vi "Dashboard Main.vi"() -> ()   [LabVIEW 2017]
uses:
  <vilib>/Utility/miscctls.llb/LVRowAndColumnTypeDef.ctl
  <vilib>/event_ctls.llb/eventvkey.ctl
  <vilib>/Rock Robotics/Network Tables/NT Read Numeric Array.vi
  <vilib>/Rock Robotics/WPI/Dashboard/WPI_DashboardLogging Global.vi
  <vilib>/Rock Robotics/Network Tables/NT Write Boolean.vi
panel:
  in  "Camera Settings Right":T1={"Frame Rate"=30, "Compression"=30, "Size"=1, "DB Camera Config"=FALSE} {"Frame Rate" scale=1.0..30.0; "Compression" scale=100.0..-1.0; "Size" items=["640x480", "320x240", "160x120"]}
  in  "Camera Name Right":string(combo)="No Camera Selection"
  out "Camera Info":cluster{"Mbps LED":bool, "Mbps":dbl, "fps":dbl} {"fps" format="%#.1g"; "Mbps" format="%#.1g"}
  in  "Camera Settings":T1={"Frame Rate"=30, "Compression"=30, "Size"=1, "DB Camera Config"=FALSE} {"Frame Rate" scale=1.0..30.0; "Compression" scale=100.0..-1.0; "Size" items=["640x480", "320x240", "160x120"]}
  in  "TCP":refnum<k5>
  in  "Rec Mode":enum32{"Stop", "Record", "Playback"}(radio)
  out "Robot IP":string
  out "Image Message":string="Timeout in Camera Communications"
  in  "Dashboard Tab":T2(tab)
  out "Game Data":string
  in  "Select test":string(combo)="with_delay"
  out "NT Connection":bool
  out "MotorChart R":cluster{"Numeric":dbl, "Numeric":dbl}(graph)
  out "MotorChart L":cluster{"Numeric":dbl, "Numeric":dbl}(graph)
  out "MotorSliders R":cluster{"MotorSlide1":dbl, "MotorSlide2":dbl} {"MotorSlide2" scale=-1.0..1.0 scale format="%#_2e"; "MotorSlide1" scale=-1.0..1.0 scale format="%#_2e"}
  out "MotorSliders L":cluster{"MotorSlide1":dbl, "MotorSlide2":dbl} {"MotorSlide2" scale=-1.0..1.0 scale format="%#_2e"; "MotorSlide1" scale=-1.0..1.0 scale format="%#_2e"}
  out "JS1 Z":dbl(slide) scale=-1.0..1.0 scale format="%#_2e"
  out "JS1 Graph":cluster{"X":dbl, "Y":dbl}[](graph)
  out "JS1 Buttons":T3
  out "JS2 Z":dbl(slide) scale=-1.0..1.0 scale format="%#_2e"
  out "JS2 Graph":cluster{"X":dbl, "Y":dbl}[](graph)
  out "JS2 Buttons":T3
  out "Mode":T4(ring)=enum."Auto Disabled"
  out "Camera Image Right":T5(plugin-control)
  in  "DB/String 9":string
  in  "DB/String 8":string
  in  "DB/String 7":string
  in  "DB/String 6":string
  in  "DB/String 5":string
  in  "DB/String 4":string
  in  "DB/String 3":string
  in  "DB/String 2":string
  in  "DB/String 1":string
  in  "DB/String 0":string
  in  "DB/Slider 0":dbl(slide) scale=0.0..5.0
  in  "DB/Slider 1":dbl(slide) scale=0.0..5.0
  in  "DB/Slider 2":dbl(slide) scale=0.0..5.0
  in  "DB/Slider 3":dbl(slide) scale=0.0..5.0
  out "DB/LED 3":bool
  out "DB/LED 2":bool
  out "DB/LED 1":bool
  out "DB/LED 0":bool
  in  "DB/Button 3":bool
  in  "DB/Button 2":bool
  in  "DB/Button 1":bool
  in  "DB/Button 0":bool caption="New Name"
  in  "Position":string(combo)="L"
  in  "A second driver":bool
  in  "Select Auto":string(combo)="with_delay"
  in  "Test Slider":dbl(slide) scale=0.0..100.0 scale format="%#_3g"
  in  "On/Off":bool caption="Solenoid"
  in  "Test Name":u16(ring) items=["Select the test to run..."]
  in  "Test Tree":string(tree)
  in  "Motor":cluster{"Value":dbl, "Enable":bool} {"Value" scale=-1.0..1.0 scale format="%#_3g"}
  out "Progress":T6 {"Test Progress" scale=0.0..100.0}
  in  "Rev/Fwd":cluster{"Forward":bool, "Reverse":bool}
  in  "Test Ring":u16(ring) items=["Monochrome", "Color"]
  out "Cmd Status":string
  in  "Execute Command":bool
  in  "Command Params":string[][](table)
  in  "Command Selection":i32(listbox)
  in  "CheckList":i32(listbox)
  out "Tree":string(tree)
  out "Camera Image":T5(plugin-control)
  out "Background":bool
  in  "Camera Name":string(combo)="Camera"
  # "HW"
  # "HW"
  # "Front"
  # "Joysticks"
  # "Left"
  # "Right"
  # "Back"
  # "This string shows the position of the switch and the scale,\nthe first letter is our switch,the second is the scale,\nand the last one is OPFOR's switch."
  # "This tab is a great place for autonomous settings and robot-specific values.\nPlace controls and indicators inside this tab and match name to\nDashboard Variables on robot. You can also delete this comment."
  # "This auto selector is not used any more,\nbecause the combo button seldom works."
  # "If you press that, the teleop will\nchange to the dual driver mode.\n(DISABLED NOW,always in dual mode)"
  # "Which tells you the actual position\nof the robot when you change it\nwith your other alliance member."
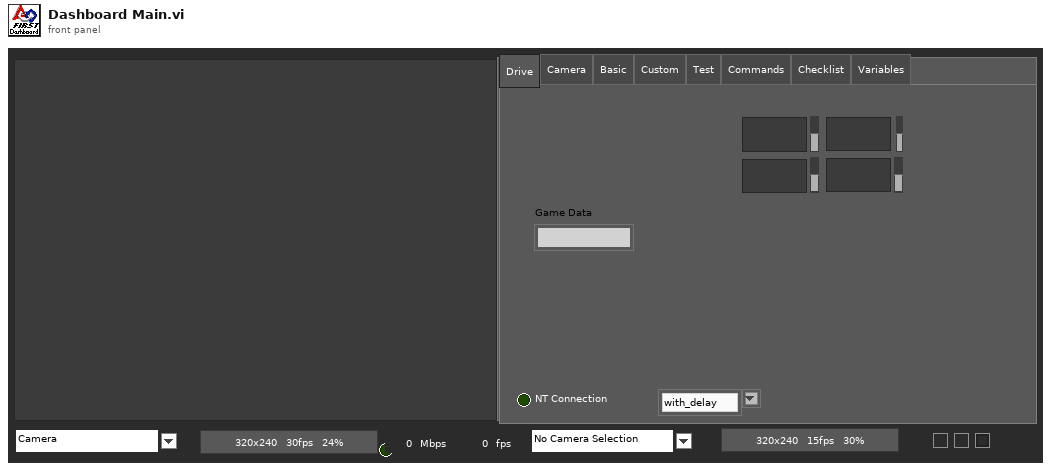
[diagram p1: front panel]
types:
  T1 = cluster{"Frame Rate":i32, "Compression":i32, "Size":u16, "DB Camera Config":bool}
  T2 = enum32{"Drive", "Camera", "Basic", "Custom", "Test", "Commands", "Checklist", "Variables"}
  T3 = cluster{bool, bool, bool, bool, bool, bool, bool, bool, bool, bool, bool, bool}
  T4 = enum8{"Tele-Op Disabled", "Tele-Op Enabled", "Auto Disabled", "Auto Enabled", "Test Disabled", "Test Enabled", "Disconnected", "No Code", "E-Stop"}
  T5 = typedef "IMAQ Image.ctl" = refnum<image>
  T6 = cluster{"Test Progress":u8, "Test Progress Text":string}
  T7 = cluster{"Save Path":path, "Interval (s)":dbl, "Keep":i32}
  T8 = typedef "Image Type" = u32
  T9 = cluster{"IDs":cluster{"RPC field ID":u16, "Unique ID":u16}, "String":string}
  T10 = cluster{"Error Strings":string, "Disable Counts":cluster{u16, u16}, "Rail Faults":cluster{u16, u16, u16}, "Robot IP":string, "DB Mode":u8, "Event Info":cluster{"Name":string, "Type":u8, "Number":u16, "Replay":u8}}
  T11 = cluster{"Storage":cluster{"Disk Free":u64, "RAM Block":u32, "RAM free":u32}, "CPU Utilization":cluster{"CPU % ISR":sgl, "CPU % Time Crit":sgl, "CPU % Timed Str":sgl, "CPU % High":sgl, "CPU % Above":sgl, "CPU % Normal":sgl, "CPU % Low":sgl}, "CAN":cluster{"% Bus Utilization":sgl, "Bus Off Cnt":u32, "TX_FIFO Full Cnt":u32, "Receive Error Cnt":u8, "Transmit Error Cnt":u8}, "HID":cluster{"HID Outputs":u32, "Rumble Low":u16, "Rumble High":u16}[]}
  T12 = cluster{"Status bits":cluster{"Test Mode":bool, "Autonomous":bool, "Enabled":bool, "Code Start":bool, "Brownout":bool, "Reserved 2":bool, "Reserved 3":bool, "E-Stop":bool}, "Code Trace":cluster{"Disabled":bool, "TeleOp":bool, "Auto":bool, "Test":bool}, "Controller Type":enum16{"unknown", "cRIO", "roboRio"}, "Code?":enum16{"unknown", "noCode", "code"}, "Battery V":dbl}
  T13 = cluster{"Control Bits":cluster{"TestMode":bool, "Autonomous":bool, "Enabled":bool, "FMS Present":bool, bool, bool, bool, "E-Stop":bool}, "Team Station ":u8, "Countdown":sgl, "Joystick Values":cluster{"Axes":dbl[], "Buttons":bool[], "POVs":i16[]}[]}
  T14 = cluster{"Axes":dbl[], "Buttons":bool[], "POVs":i16[]}[]
  T15 = cluster{"Axes":dbl[], "Buttons":bool[], "POVs":i16[]}
  T16 = cluster{"Buttons[0]":bool, "Buttons[1]":bool, "Buttons[2]":bool, "Buttons[3]":bool, "Buttons[4]":bool, "Buttons[5]":bool, "Buttons[6]":bool, "Buttons[7]":bool, "Buttons[8]":bool, "Buttons[9]":bool, "Buttons[10]":bool, "Buttons[11]":bool}
  T17 = cluster{"Camera Image":refnum<vi>, "Dashboard Tab":refnum<vi>, "Background":refnum<vi>, "Rec Mode":refnum<vi>, "Test Slider":refnum<vi>, "On/Off ":refnum<vi>, "Test Ring":refnum<vi>, "Rev/Fwd":refnum<vi>, "Test Name":refnum<vi>, "Motor":refnum<vi>, "Progress":refnum<vi>, "CheckList":refnum<vi>, "Tree":refnum<vi>, "Test Tree":refnum<vi>, "Command Params":refnum<vi>, "Command Selection":refnum<vi>, "Execute Command":refnum<vi>, "Cmd Status":refnum<vi>, "Camera Settings":refnum<vi>, "Camera Name":refnum<vi>, "Camera Info":refnum<vi>, "Camera Settings Right":refnum<vi>, "Camera Name Right":refnum<vi>, "Camera Image Right":refnum<vi>}
  T18 = cluster{"Camera Name":string, string, "Saved DB Images Info":cluster{"Save Path":path, "Interval (s)":dbl, "Keep":i32}}
  T19 = cluster{"Camera Name Right":string, string, "Saved DB Images Info":cluster{"Save Path":path, "Interval (s)":dbl, "Keep":i32}}
  T20 = cluster{"Operation":enum16{"Update", "Clear"}, "Color Box":u32}[]
  T21 = typedef "eventvkey.ctl" = enum16{"ASCII", "Enter", "Return", "Shift", "Ctrl", "Alt", "Cmd", "Opt", "Caps", "NumLock", "Clear", "Break", "Up", "Down", "Left", "Right", "Insert", "Delete", "Home", "End", "PageUp", "PageDown", "Escape", "Help", "Pause", "ScrollLock", "F1", "F2", "F3", "F4", "F5", "F6", "F7", "F8", "F9", "F10", "F11", "F12", "F13", "F14", "F15", "F16", "F17", "F18", "F19", "F20", "F21", "F22", "F23", "F24", "Play", "VolumeUp", "VolumeDown", "Mute", "Two Byte Char"}
  T22 = cluster{"Image Size":bool, "Image Type":bool, "Pixel Value":bool, "ROI Information":bool, "Zoom Factor":bool}
  T23 = cluster{"Operation":enum16{"Update", "Clear"}, "Color Box":u32}
  T24 = typedef "LVRowAndColumnTypeDef.ctl" = cluster{"Row":i32, "Column":i32}
  T25 = cluster{"Shift":bool, "Ctrl":bool, "Alt":bool, "Cmd":bool, "Opt":bool}
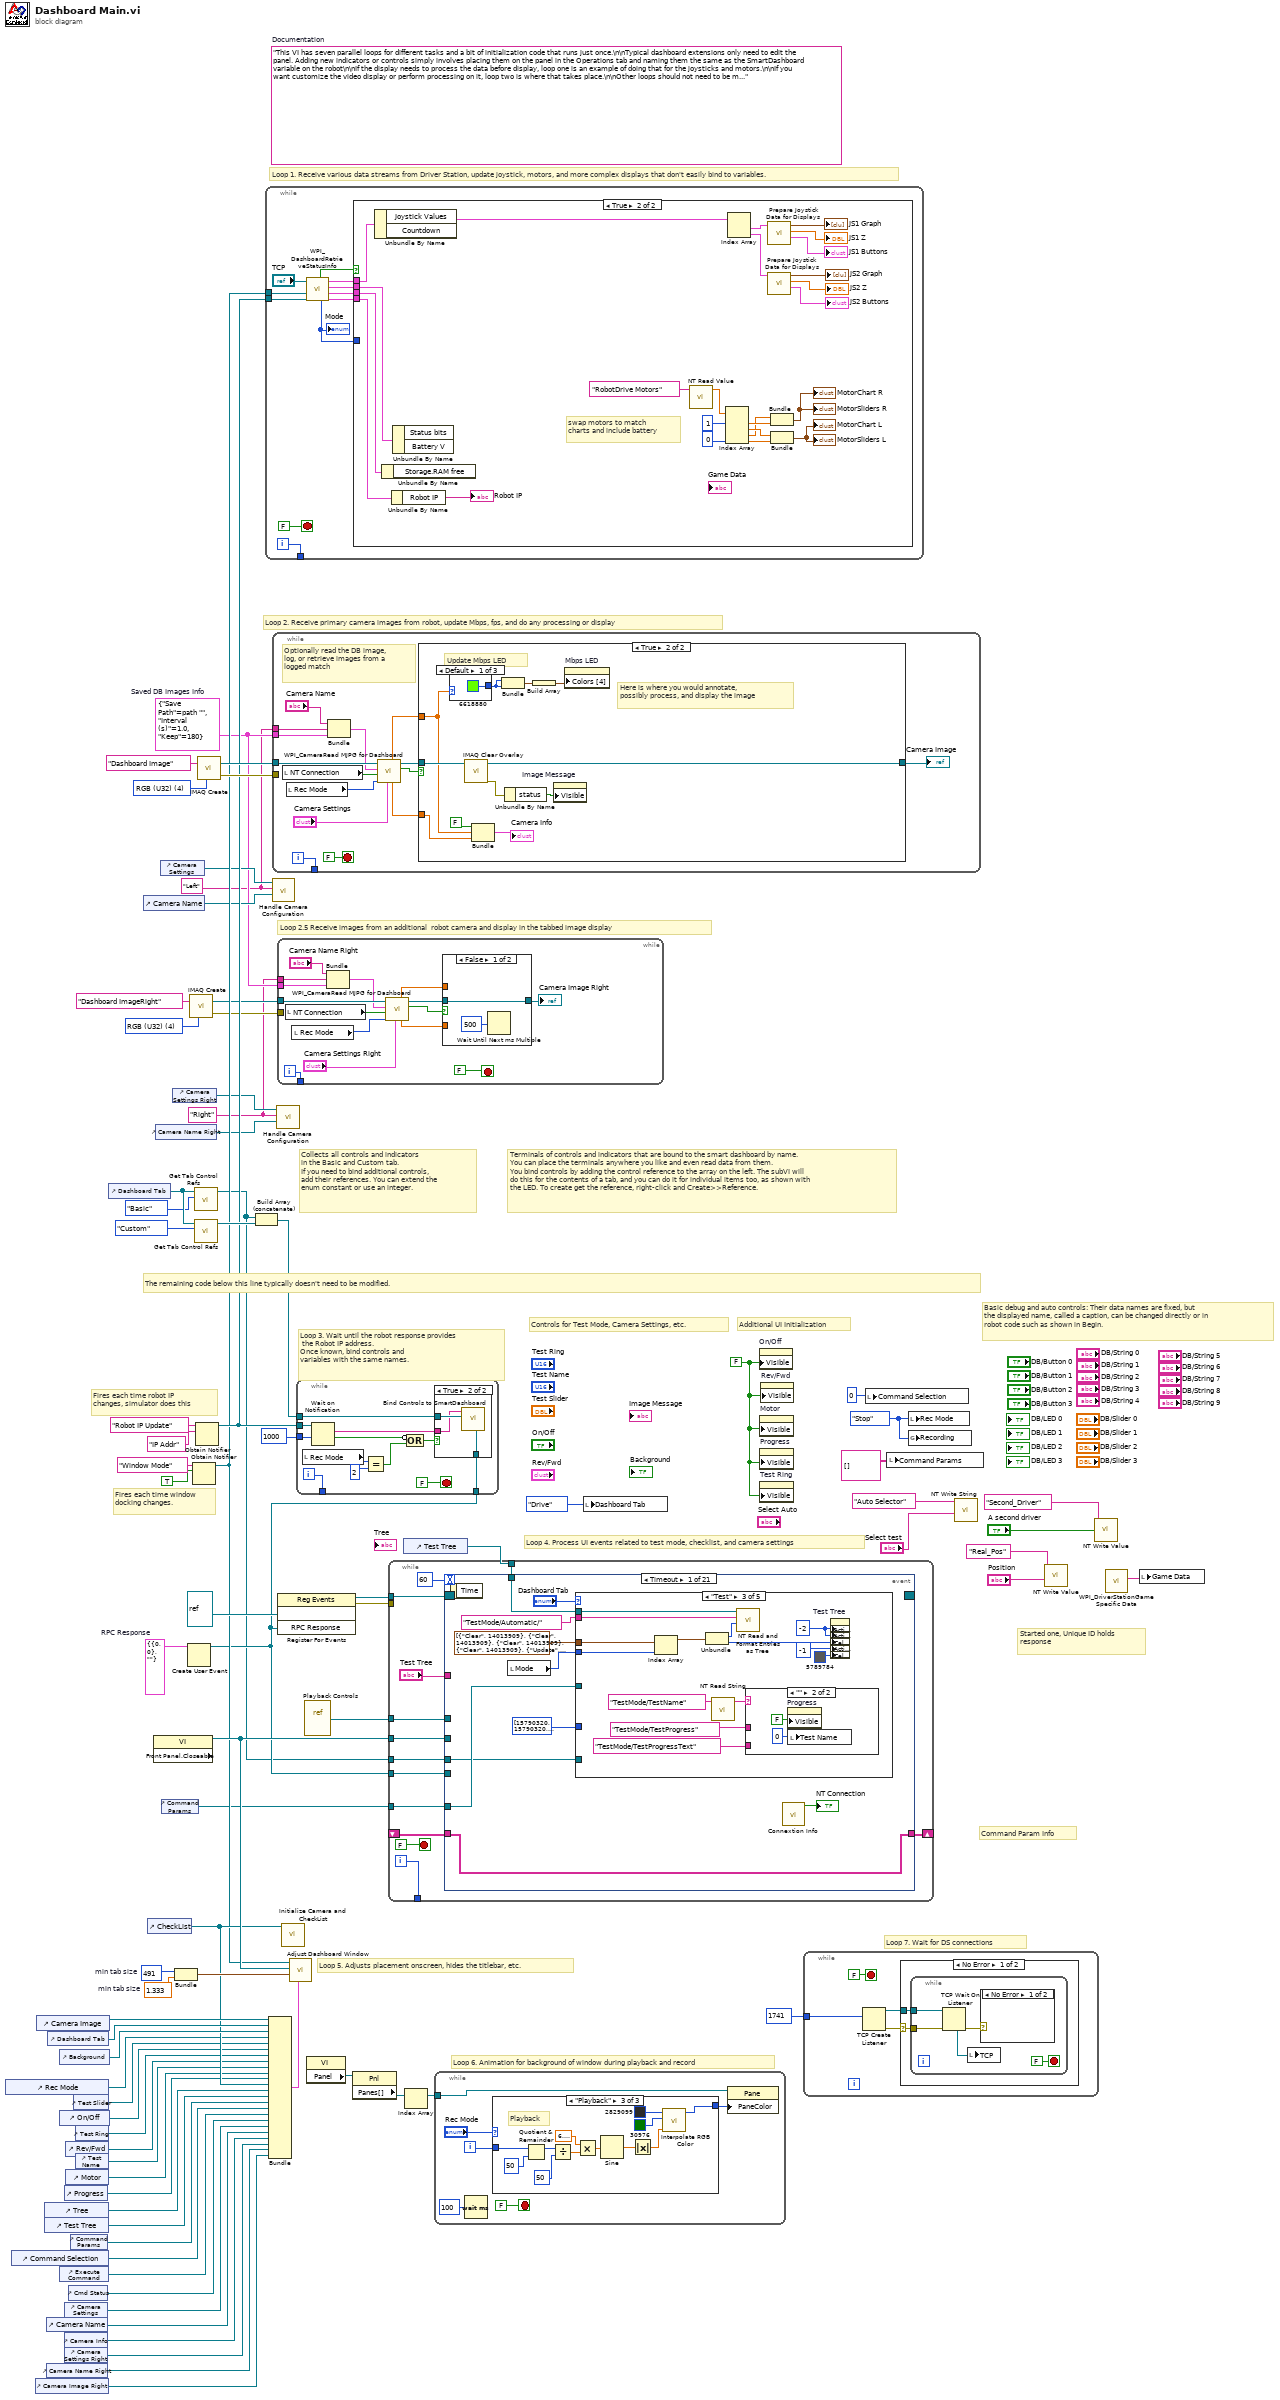
[diagram p0: block diagram]
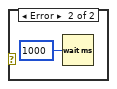
[diagram p3: hidden frame]
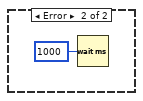
[diagram p4: hidden frame]
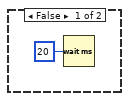
[diagram p5: hidden frame]
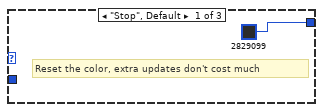
[diagram p6: hidden frame]
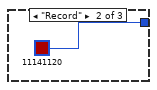
[diagram p7: hidden frame]
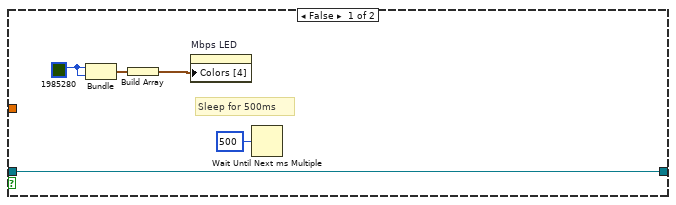
[diagram p9: hidden frame]
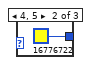
[diagram p10: hidden frame]
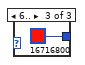
[diagram p11: hidden frame]
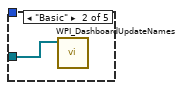
[diagram p13: hidden frame]
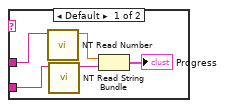
[diagram p14: hidden frame]
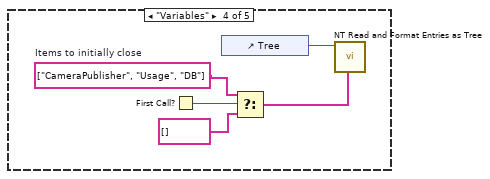
[diagram p15: hidden frame]
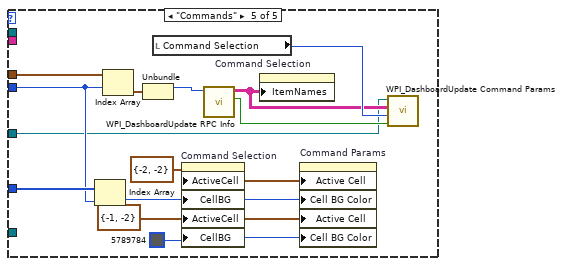
[diagram p16: hidden frame]
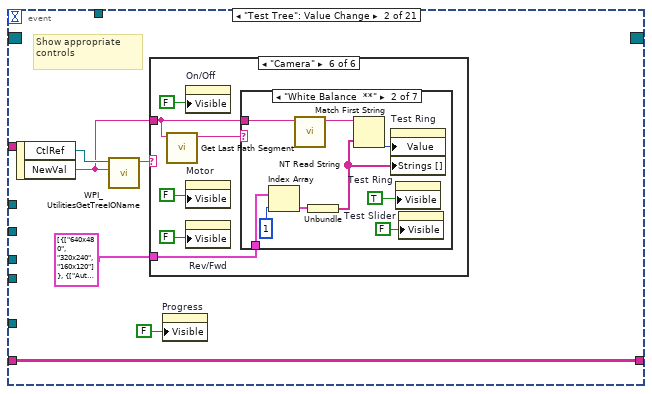
[diagram p17: hidden frame]
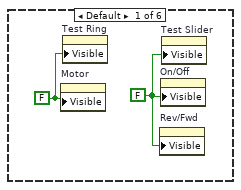
[diagram p18: hidden frame]
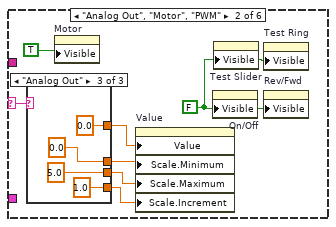
[diagram p19: hidden frame]
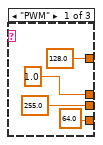
[diagram p20: hidden frame]
diagram:
  w9 = T7 {"Save Path"=path "", "Interval (s)"=1.0, "Keep"=180}  # Saved DB Images Info
  w8 = "Right"
  w7 = "Left"
  w19 = T8 4 items=["Grayscale (U8)", "Grayscale (I16)", "Grayscale (SGL)", "Complex (CSG)", "RGB (U32)", "HSL (U32)", "RGB (U64)"] ("Image Type")
  w34 = T9 {"IDs"={"RPC field ID"=0, "Unique ID"=0}, "String"=""}  # RPC Response
  w57 = 491  # min tab size
  w56 = 1.333  # min tab size
  w64 = enum32{"Stop", "Record", "Playback"}."Stop" ("Rec Mode")
  w41 = FALSE ("Visible")
  (unwired) "This VI has seven parallel loops for different tasks and a bit of initialization code that runs just once.\n\nTypical dashboard extensions only need to edit the panel. Adding new indicators or controls simply involves placing them on the panel in the Operations tab and naming them the same as the SmartDashboard variable on the robot\n\nIf the display needs to process the data before display, loop one is an example of doing that for the joysticks and motors.\n\nIf you want customize the video display or perform processing on it, loop two is where that takes place.\n\nOther loops should not need to be modified. They are pretty standard, and document the task they perform."  # Documentation
  w81 = T8 4 items=["Grayscale (U8)", "Grayscale (I16)", "Grayscale (SGL)", "Complex (CSG)", "RGB (U32)", "HSL (U32)", "RGB (U64)"] ("Image Type")
  # "Loop 2.5 Receive images from an additional  robot camera and display in the tabbed image display"
  # "Command Param Info"
  # "Started one, Unique ID holds\nresponse"
  # "Loop 7. Wait for DS connections"
  # "Basic debug and auto controls: Their data names are fixed, but\nthe displayed name, called a caption, can be changed directly or in\nrobot code such as shown in Begin."
  # "Controls for Test Mode, Camera Settings, etc."
  # "Additional UI Initialization"
  # "Loop 6. Animation for background of window during playback and record"
  # "Fires each time robot IP\nchanges, simulator does this"
  # "Fires each time window\ndocking changes."
  # "Collects all controls and indicators\nin the Basic and Custom tab.\nIf you need to bind additional controls,\nadd their references. You can extend the\nenum constant or use an integer."
  # "The remaining code below this line typically doesn't need to be modified."
  # "Loop 4. Process UI events related to test mode, checklist, and camera settings"
  # "Terminals of controls and indicators that are bound to the smart dashboard by name.\nYou can place the terminals anywhere you like and even read data from them.\nYou bind controls by adding the control reference to the array on the left. The subVI will\ndo this for the contents of a tab, and you can do it for individual items too, as shown with\nthe LED. To create get the reference, right-click and Create>>Reference."
  # "Loop 3. Wait until the robot response provides\n the Robot IP address.\nOnce known, bind controls and\nvariables with the same names."
  # "Loop 5. Adjusts placement onscreen, hides the titlebar, etc."
  # "Loop 1. Receive various data streams from Driver Station, update joystick, motors, and more complex displays that don't easily bind to variables."
  # "Loop 2. Receive primary camera images from robot, update Mbps, fps, and do any processing or display"
  n1 = control-ref of="Rec Mode"() -> (w47:refnum<vi>)
  n2 = control-ref of="Command Selection"() -> (w33:refnum<vi>)
  n3 = control-ref of="Camera Image Right"() -> (w12:refnum<vi>)
  n4 = control-ref of="Camera Image"() -> (w59:refnum<vi>)
  n5 = control-ref of="Tree"() -> (w51:refnum<vi>)
  n6 = control-ref of="Test Tree"() -> (w50:refnum<vi>)
  n7 = control-ref of="Camera Name"() -> (w24:refnum<vi>)
  n8 = control-ref of="Camera Name Right"() -> (w13:refnum<vi>)
  n9 = control-ref of="Dashboard Tab"() -> (w58:refnum<vi>)
  n10 = control-ref of="Execute Command"() -> (w35:refnum<vi>)
  n11 = control-ref of="Background"() -> (w54:refnum<vi>)
  n12 = control-ref of="On/Off"() -> (w45:refnum<vi>)
  n13 = control-ref of="Progress"() -> (w42:refnum<vi>)
  n14 = control-ref of="Camera Settings"() -> (w25:refnum<vi>)
  n15 = control-ref of="Camera Info"() -> (w23:refnum<vi>)
  n16 = control-ref of="Camera Settings Right"() -> (w14:refnum<vi>)
  n17 = control-ref of="Rev/Fwd"() -> (w43:refnum<vi>)
  n18 = control-ref of="Motor"() -> (w48:refnum<vi>)
  n19 = control-ref of="Cmd Status"() -> (w29:refnum<vi>)
  n20 = control-ref of="Command Params"() -> (w36:refnum<vi>)
  n21 = control-ref of="Test Slider"() -> (w46:refnum<vi>)
  n22 = control-ref of="Test Ring"() -> (w44:refnum<vi>)
  n23 = control-ref of="Test Name"() -> (w49:refnum<vi>)
  n24 = control-ref of="Dashboard Tab"() -> (w62:refnum<vi>)
  n25 = control-ref of="Camera Name"() -> (w26:refnum<vi>)
  n26 = control-ref of="CheckList"() -> (w52:refnum<vi>)
  n27 = property class="VI" props=["Front Panel.Closeable"]() -> (reference out=w63:refnum<vi>)  [unwired: 2 in, 2 out]
  n28 = control-ref of="Camera Name Right"() -> (w15:refnum<vi>)
  n29 = control-ref of="Camera Settings"() -> (w27:refnum<vi>)
  n30 = control-ref of="Command Params"() -> (w28:refnum<vi>)
  n31 = control-ref of="Camera Settings Right"() -> (w16:refnum<vi>)
  n32 = Bundle("min tab size"=w57, "min tab size"=w56) -> (w55:cluster{"min tab size":i32, "min tab size":dbl})  [unwired: 1 in]
  n33 = Create User Event(user event datatype=w34) -> (user event=w30:refnum<user-event>)  [unwired: 1 in, 1 out]
  n34 = call "IMAQ Create"("Image Name"="Dashboard ImageRight", "Image Type"=w19) -> ("New Image"=w18:T5, "error out"=w17:errorcluster)  [unwired: 2 in, 1 out]
  n35 = Obtain Notifier(name (unnamed)="Window Mode", notification data type=TRUE) -> (notifier out=w39:refnum<notifier>)  [unwired: 2 in, 2 out]
  n36 = call <vilib>:"Get Tab Control Refs.vi"("Page Index"=T2."Basic" ("Dashboard Tab"), "TabControl in"=w62) -> ("ControlsOnPage"=w22:refnum<vi>[])  [unwired: 9 in]
  n37 = call <vilib>:"Get Tab Control Refs.vi"("Page Index"=T2."Custom" ("Dashboard Tab"), "TabControl in"=w62) -> ("ControlsOnPage"=w61:refnum<vi>[])  [unwired: 9 in]
  n38 = Obtain Notifier(name (unnamed)="Robot IP Update", notification data type="IP Addr" ("name (unnamed)")) -> (notifier out=w40:refnum<notifier>)  [unwired: 2 in, 2 out]
  n39 = call "IMAQ Create"("Image Name"="Dashboard Image", "Image Type"=w81) -> ("New Image"=w79:T5, "error out"=w78:errorcluster)  [unwired: 2 in, 1 out]
  n40 = Build Array (concatenate)(w22, w61) -> (w60:refnum<vi>[])
  n41 = while {
    tunnel: [w91] -> _
    tunnel: w40 -> [w85]
    tunnel: w39 -> [w82]
    i -> [w91]
    stop <- FALSE stop-if-true
    n42 = call <vilib>:"WPI_DashboardRetrieveStatusInfo.vi"("Binding Refnum"=w85, "Window Mode Notifier"=w82, "TCP Cnx"="TCP") -> ("Power and Errors"=w86:T10, "Robot Metrics"=w89:T11, "Status Info"=w90:T12, "Control Info"=w87:T13, "Robot Mode"=w84:T4, "Process?"=w88:bool)  [unwired: 3 in]
    "Mode" <- w84
    n43 = case shown="True" w88 {
      tunnel: w90 -> [_ w117]
      tunnel: w89 -> [_ w116]
      tunnel: w87 -> [_ w115]
      tunnel: w86 -> [_ w114]
      tunnel: w84 -> [_ _]
      frame False {
        n44 = Wait (ms)(milliseconds to wait=u32 20) -> ()  [unwired: 1 out]
      }
      frame True {
        # "swap motors to match\ncharts and include battery"
        n45 = Unbundle By Name(w115) -> ("Joystick Values"=w105:T14)  [unwired: 1 out]
        n46 = Unbundle By Name(w116) -> ()  [unwired: 1 out]
        n47 = Unbundle By Name(w114) -> ("Robot IP"=→"Robot IP":string)
        n48 = Unbundle By Name(w117) -> ()  [unwired: 2 out]
        n49 = call-poly <vilib>:"NT Read Value.vi"("Name"="RobotDrive Motors") -> ("Numeric Array"=w95:dbl[])  [unwired: 9 in, 1 out]
        n50 = Index Array(array=w95, index #1=1, index #4=0) -> (element #1=w109:dbl, element #2=w110:dbl, element #3=w108:dbl, element #4=w113:dbl)  [unwired: 2 in]
        n51 = Index Array(array=w105) -> (element #1=w104:T15, element #2=w100:T15)  [unwired: 2 in]
        n52 = call "Prepare Joystick Data for Displays.vi"("Joystick Values"=w100) -> ("Buttons"=→"JS2 Buttons":T16, "Z Axis"=→"JS2 Z":dbl, "Cartesian Data"=→"JS2 Graph":cluster{"X axis":dbl, "X axis":dbl}[])  [unwired: 8 in]
        n53 = call "Prepare Joystick Data for Displays.vi"("Joystick Values"=w104) -> ("Buttons"=→"JS1 Buttons":T16, "Z Axis"=→"JS1 Z":dbl, "Cartesian Data"=→"JS1 Graph":cluster{"X axis":dbl, "X axis":dbl}[])  [unwired: 8 in]
        n54 = Bundle("Numeric"=w108, "Numeric"=w109) -> (→"MotorChart R" →"MotorSliders R":cluster{"Numeric":dbl, "Numeric":dbl})  [unwired: 1 in]
        n55 = Bundle("Numeric"=w110, "Numeric"=w113) -> (→"MotorChart L" →"MotorSliders L":cluster{"Numeric":dbl, "Numeric":dbl})  [unwired: 1 in]
      }
    }
  }
  n56 = Bundle("Camera Image"=w59, "Dashboard Tab"=w58, "Background"=w54, "Rec Mode"=w47, "Test Slider"=w46, "On/Off"=w45, "Test Ring"=w44, "Rev/Fwd"=w43, "Test Name"=w49, "Motor"=w48, "Progress"=w42, "CheckList"=w52, "Tree"=w51, "Test Tree"=w50, "Command Params"=w36, "Command Selection"=w33, "Execute Command"=w35, "Cmd Status"=w29, "Camera Settings"=w25, "Camera Name"=w24, "Camera Info"=w23, "Camera Settings Right"=w14, "Camera Name Right"=w13, "Camera Image Right"=w12) -> (w53:T17)  [unwired: 1 in]
  n57 = call "Handle Camera Configuration.vi"("CameraNameRef"=w26, "Display Name"=w7, "ClusterRef"=w27) -> ()  [unwired: 9 in]
  n58 = while {
    tunnel: w79 -> [w130]
    tunnel: w78 -> [_]
    tunnel: [w131] -> _
    tunnel: w9 -> [w121]
    tunnel: w7 -> [w118]
    i -> [w131]
    stop <- FALSE stop-if-true
    # "Optionally read the DB image,\nlog, or retrieve images from a\nlogged match"
    n59 = local read "NT Connection"() -> (w122:bool)
    n60 = local read "Rec Mode"() -> (w126:enum32{"Stop", "Record", "Playback"})
    n61 = Bundle("Camera Name"="Camera Name", w118, "Saved DB Images Info"=w121) -> (w120:T18)  [unwired: 1 in]
    n62 = call <vilib>:"WPI_CameraRead MJPG for Dashboard.vi"("Camera Settings"="Camera Settings", "Rec Mode"=w126, "NT Connection"=w122, "Capture Info"=w120, "Refnum in"=w130) -> ("Active"=w128:bool, "Refnum out"=w129:T5, "FPS"=w127:dbl, "Bandwidth (Mbps)"=w125:dbl)  [unwired: 3 in]
    n63 = case shown="True" w128 {
      tunnel: w129 -> [w133 w144]
      tunnel: w125 -> [_ w141]
      tunnel: w127 -> [_ w142]
      tunnel: [w133 w138] -> w123
      frame False {
        w135 = u32 1985280 ("Color Box")
        # "Sleep for 500ms"
        n64 = Bundle("Color Box"=w135, "Color Box"=w135) -> (w136:cluster{"Color Box":u32, "Color Box":u32})  [unwired: 1 out]
        n65 = Build Array(w136) -> (w134:cluster{"Color Box":u32, "Color Box":u32}[])
        n66 = property on="Mbps LED" class="Bool (strict)"("Colors [4]"=w134) -> ()  [unwired: 2 in, 2 out]
        n67 = Wait Until Next ms Multiple(millisecond multiple=u32 500) -> ()  [unwired: 1 out]
      }
      frame True {
        # "Here is where you would annotate,\npossibly process, and display the image"
        # "Update Mbps LED"
        n68 = case shown="Default" w141 {
          tunnel: [u32 6618880 ("Color Box") u32 16776722 ("Color Box") u32 16716800 ("Color Box")] -> w145
          frame Default {
          }
          frame 4, 5 {
          }
          frame 6.. {
          }
        }
        n69 = call "IMAQ Clear Overlay"("Image"=w144) -> ("error out"=w147:errorcluster, "Image Out"=w138:T5)  [unwired: 2 in, 7 out]
        n70 = Bundle(FALSE, "Bandwidth (Mbps)"=w141, "FPS"=w142) -> (→"Camera Info":cluster{bool, "Bandwidth (Mbps)":dbl, "FPS":dbl})  [unwired: 1 in]
        n71 = Bundle("Color Box"=w145, "Color Box"=w145) -> (w146:cluster{"Color Box":u32, "Color Box":u32})  [unwired: 1 out]
        n72 = Unbundle By Name(w147) -> ("status"=w148:bool)
        n73 = Build Array(w146) -> (w143:cluster{"Color Box":u32, "Color Box":u32}[])
        n74 = property on="Image Message" class="Str"("Visible"=w148) -> ()  [unwired: 2 in, 2 out]
        n75 = property on="Mbps LED" class="Bool (strict)"("Colors [4]"=w143) -> ()  [unwired: 2 in, 2 out]
      }
    }
    "Camera Image" <- w123
  }
  n76 = call "Handle Camera Configuration.vi"("CameraNameRef"=w15, "Display Name"=w8, "ClusterRef"=w16) -> ()  [unwired: 9 in]
  n77 = while {
    tunnel: w18 -> [w166]
    tunnel: w17 -> [_]
    tunnel: [w161] -> _
    tunnel: w9 -> [w155]
    tunnel: w8 -> [w152]
    i -> [w161]
    stop <- FALSE stop-if-true
    n78 = local read "NT Connection"() -> (w156:bool)
    n79 = local read "Rec Mode"() -> (w165:enum32{"Stop", "Record", "Playback"})
    n80 = Bundle("Camera Name Right"="Camera Name Right", w152, "Saved DB Images Info"=w155) -> (w154:T19)  [unwired: 1 in]
    n81 = call <vilib>:"WPI_CameraRead MJPG for Dashboard.vi"("Camera Settings"="Camera Settings Right", "Rec Mode"=w165, "NT Connection"=w156, "Capture Info"=w154, "Refnum in"=w166) -> ("Active"=w160:bool, "Refnum out"=w163:T5, "FPS"=w158:dbl, "Bandwidth (Mbps)"=w159:dbl)  [unwired: 3 in]
    n82 = case shown="False" w160 {
      tunnel: w163 -> [w167 w169]
      tunnel: w159 -> [_ _]
      tunnel: w158 -> [_ _]
      tunnel: [w167 w169] -> w157
      frame False {
        n83 = Wait Until Next ms Multiple(millisecond multiple=u32 500) -> ()  [unwired: 1 out]
      }
      frame True {
      }
    }
    "Camera Image Right" <- w157
  }
  n84 = register-events(refnum<vi> refnum, w30) -> (reference out=w68:refnum<event-registration>, error out=w67:errorcluster)  [unwired: 2 in]
  n85 = call "Initialize Camera and CheckList.vi"("ListBox in"=w52) -> ()  [unwired: 11 in]
  n86 = call "Adjust Dashboard Window.vi"("Sizing Refnums"=w53, "Size Constraints"=w55, "VI"=w63, "WIn Mode"=w39) -> ()  [unwired: 8 in]
  n87 = while {
    tunnel: w60 -> [w181]
    tunnel: w40 -> [w179]
    tunnel: [w177] -> _
    tunnel: u32 1000 ("milliseconds to wait") -> [w176]
    tunnel: w30 -> [w170]
    i -> [w177]
    stop <- FALSE stop-if-true
    n88 = local read "Rec Mode"() -> (w172:enum32{"Stop", "Record", "Playback"})
    n89 = Wait on Notification(notifier=w179, timeout in ms (-1)=w176) -> (notification=w178:string, timed out?=w174:bool)  [unwired: 2 in, 2 out]
    n90 = Equal?(x=w172, y=u16 2 ("Rec Mode")) -> (x = y?=w173:bool)
    n91 = Compound Arithmetic op=OR(invert w174, w173) -> (w175:bool)
    n92 = case shown="True" w175 {
      tunnel: w181 -> [_ w184]
      tunnel: w178 -> [_ w183]
      tunnel: w170 -> [_ w182]
      frame False {
      }
      frame True {
        n93 = call <vilib>:"Bind Controls to SmartDashboard.vi"("RPC ref"=w182, "Bound Control Refs"=w184, "Server IP Address"=w183) -> ()  [unwired: 9 in]
      }
    }
  }
  n94 = vi-ref "Playback Controls.vi"() -> (w69:refnum<vi>)
  n95 = property class="VI"() -> ("Panel"=w71:refnum<vi>)  [unwired: 2 in, 2 out]
  n96 = property class="Pnl"(reference=w71) -> ("Panes[]"=w72:refnum<vi>[])  [unwired: 1 in, 2 out]
  n97 = control-ref of="Test Tree"() -> (w73:refnum<vi>)
  n98 = while {
    tunnel: [w194] -> _
    tunnel: w73 -> [w193]
    tunnel: w69 -> [w192]
    tunnel: w68 -> [w191]
    tunnel: w67 -> [_]
    tunnel: w63 -> [w190]
    tunnel: w30 -> [w189]
    tunnel: w28 -> [w188]
    shift-right: [w187] -> _
    shift-left: _ -> [w186]
    tunnel: w22 -> [w185]
    i -> [w194]
    stop <- FALSE stop-if-true
    n99 = event shown="[0] Timeout" {
      selector: w191 -> [_ _ _ _ _ _ _ _ _ _ _ _ _ _ _ _ _ _ _ _ _]
      dyn-events: [_ _ _ _ _ _ _ _ _ _ _ _ _ _ _ _ w454 _ _ _ _] -> _
      timeout: u32 60 ("milliseconds to wait") -> [_ _ _ _ _ _ _ _ _ _ _ _ _ _ _ _ _ _ _ _ _]
      tunnel: w193 -> [w206 _ _ _ _ _ _ _ _ _ _ _ _ _ _ _ _ _ _ _ _]
      tunnel: "Test Tree" -> [_ _ _ _ _ _ _ _ _ _ _ w421 w429 w431 w435 w443 _ _ _ _ _]
      tunnel: w192 -> [_ _ _ _ _ _ _ _ _ _ _ _ _ _ _ _ w456 _ w474 _ _]
      tunnel: w190 -> [_ _ _ _ _ _ _ _ _ _ _ _ _ _ _ _ w452 _ _ _ _]
      tunnel: w189 -> [_ _ _ _ _ _ _ _ _ _ _ _ _ _ _ _ w450 _ _ _ _]
      tunnel: w188 -> [w201 _ _ _ _ _ w372 _ _ _ _ _ _ _ _ _ _ _ _ _ _]
      tunnel: [w200 w249 w351 w356 w365 w369 w370 w379 w389 w396 w408 w420 w427 w430 w434 w442 w449 w469 w471 w475 w488] -> w187
      tunnel: w186 -> [w200 w249 w351 w356 w365 w369 w370 _ _ w396 w408 w420 w427 w430 w434 w442 w449 w469 w471 w475 w488]
      tunnel: w185 -> [w198 _ _ _ _ _ _ _ _ _ _ _ _ _ _ _ _ _ _ _ _]
      event Timeout {
        n100 = event-data() -> ()  [unwired: 1 in, 1 out]
        n101 = local read "Mode"() -> (w203:T4)
        n102 = case shown="\"Test\"" "Dashboard Tab" {
          tunnel: w206 -> [_ _ w222 _ _]
          tunnel: "TestMode/Automatic/" ("Name Pattern") -> [_ _ w221 _ _]
          tunnel: T20 [{"Operation"=enum."Clear", "Color Box"=14013909}, {"Operation"=enum."Clear", "Color Box"=14013909}, {"Operation"=enum."Clear", "Color Box"=14013909}, {"Operation"=enum."Clear", "Color Box"=14013909}, {"Operation"=enum."Update", "Color Box"=14013909}, {"Operation"=enum."Update", "Color Box"=16777215}, {"Operation"=enum."Clear", "Color Box"=14013909}, {"Operation"=enum."Clear", "Color Box"=14013909}, {"Operation"=enum."Clear", "Color Box"=14013909}] -> [_ _ w214 _ w242]
          tunnel: w203 -> [_ _ w213 _ w241]
          tunnel: u32[] [15790320, 15790320, 15790320, 15790320, 16777215, 16777215, 15790320, 15790320, 15790320] -> [_ _ _ _ w247]
          tunnel: w201 -> [_ _ _ _ w235]
          tunnel: w198 -> [_ w208 _ _ _]
          frame "Custom", Default {
          }
          frame "Basic" {
            n103 = call <vilib>:"WPI_DashboardUpdateNames.vi"("Controls on Tab"=w208) -> ()  [unwired: 11 in]
          }
          frame "Test" {
            w220 = -2 ("Active Item:Row Number")
            n104 = Index Array(array=w214, index=w213) -> (element=w215:T23)
            n105 = Unbundle(w215) -> ("Operation"=w216:enum16{"Update", "Clear"}, "Color Box"=w217:u32)
            n106 = call <vilib>:"NT Read String.vi"("Name"="TestMode/TestName") -> ("String"=w211:string)  [unwired: 9 in, 1 out]
            n107 = call <vilib>:"NT Read and Format Entries as Tree.vi"("Operation"=w216, "Name Pattern"=w221, "Tree Refnum"=w222) -> ()  [unwired: 7 in, 2 out]
            n108 = case shown="\"\"" w211 {
              tunnel: "TestMode/TestProgress" ("Name") -> [w224 _]
              tunnel: "TestMode/TestProgressText" ("Name") -> [w223 _]
              frame Default {
                n109 = call <vilib>:"NT Read Number.vi"("Name"=w224) -> ("Numeric"=w225:dbl)  [unwired: 9 in, 1 out]
                n110 = call <vilib>:"NT Read String.vi"("Name"=w223) -> ("String"=w226:string)  [unwired: 9 in, 1 out]
                n111 = Bundle("Numeric"=w225, "String"=w226) -> (→"Progress":cluster{"Numeric":dbl, "String":string})  [unwired: 1 in]
              }
              frame "" {
                n112 = property on="Progress" class="Clust (strict)"("Visible"=FALSE) -> ()  [unwired: 2 in, 2 out]
                n113 = local write "Test Name"(u16 0) -> ()
              }
            }
            n114 = property on="Test Tree" class="Tree (strict)"("Active Item Row Number"=w220, "ActiveColNum"=w220, "CellBG"=w217, "Active Item Row Number"=-1 ("Active Item:Row Number"), "CellBG"=u32 5789784 ("Color Box")) -> ()  [unwired: 2 in, 2 out]
          }
          frame "Variables" {
            w232 = string[] ["CameraPublisher", "Usage", "DB"]  # Items to initially close
            n115 = First Call?() -> (First Call?: T/F=w233:bool)
            n116 = control-ref of="Tree"() -> (w234:refnum<vi>)
            n117 = Select(t=w232, s=w233, f=string[] []) -> (s? t:f=w230:string[])
            n118 = call <vilib>:"NT Read and Format Entries as Tree.vi"("Tags to  Close"=w230, "Tree Refnum"=w234) -> ()  [unwired: 8 in, 2 out]
          }
          frame "Commands" {
            w243 = u32 5789784 ("Color Box")
            w244 = T24 {"Row"=-1, "Column"=-2} ("Active Cell:Active Cell")
            w246 = T24 {"Row"=-2, "Column"=-2} ("Active Cell:Active Cell")
            n119 = Index Array(array=w247, index=w241) -> (element=w245:u32)
            n120 = Index Array(array=w242, index=w241) -> (element=w240:T23)
            n121 = Unbundle(w240) -> ("Operation"=w239:enum16{"Update", "Clear"})  [unwired: 1 out]
            n122 = local read "Command Selection"() -> (w238:i32)
            n123 = property on="Command Selection" class="MCListbox (strict)"("ActiveCell"=w246, "CellBG"=w245, "ActiveCell"=w244, "CellBG"=w243) -> ()  [unwired: 2 in, 2 out]
            n124 = call <vilib>:"WPI_DashboardUpdate RPC Info.vi"("Operation"=w239) -> ("update"=w237:bool, "commands"=w236:string[][])  [unwired: 9 in]
            n125 = property on="Command Selection" class="MCListbox (strict)"("ItemNames"=w236) -> ()  [unwired: 2 in, 2 out]
            n126 = property on="Command Params" class="Tbl (strict)"("Active Cell"=w246, "Cell BG Color"=w245, "Active Cell"=w244, "Cell BG Color"=w243) -> ()  [unwired: 2 in, 2 out]
            n127 = call <vilib>:"WPI_DashboardUpdate Command Params.vi"("Update"=w237, "NewVal"=w238, "Commands"=w236, "Param Tbl"=w235) -> ()  [unwired: 7 in, 1 out]
          }
        }
        n128 = call <vilib>:"Connextion Info.vi"() -> ("Connected"=→"NT Connection":bool)  [unwired: 10 in, 1 out]
      }
      event "Test Tree": Value Change {
        # "Show appropriate\ncontrols"
        n129 = event-data() -> ("CtlRef"=w252:refnum<vi>, "NewVal"=w250:string)  [unwired: 1 in]
        n130 = call <vilib>:"WPI_UtilitiesGetTreeIOName.vi"("NewVal"=w250, "TreeControl in"=w252) -> ("I/O Name"=w253:string)  [unwired: 9 in]
        n131 = case shown="\"Camera\"" w253 {
          selector: w253 -> [_ w260 _ w282 w291 _]
          tunnel: w250 -> [_ _ w279 w281 _ w298]
          tunnel: cluster{string[]}[] [{["640x480", "320x240", "160x120"]}, {["Auto", "Fixed indoor", "Fixed outdoor 1", "Fixed outdoor 2", "Fixed fluorescent 1", "Fixed fluorescent 2", "Hold current"]}, {["Auto", "Flicker-free 50 Hz", "Flicker-free 60 Hz", "Hold current"]}, {["None", "Prioritize frame rate", "Prioritize image quality"]}, {["Monochrome", "Color"]}] -> [_ _ _ _ _ w297]
          frame Default {
            w255 = FALSE ("Visible")
            w254 = FALSE ("Visible")
            n132 = property on="Motor" class="Clust (strict)"("Visible"=w254) -> ()  [unwired: 2 in, 2 out]
            n133 = property on="Test Ring" class="Ring (strict)"("Visible"=w254) -> ()  [unwired: 2 in, 2 out]
            n134 = property on="Rev/Fwd" class="Clust (strict)"("Visible"=w255) -> ()  [unwired: 2 in, 2 out]
            n135 = property on="On/Off" class="Bool (strict)"("Visible"=w255) -> ()  [unwired: 2 in, 2 out]
            n136 = property on="Test Slider" class="Slide (strict)"("Visible"=w255) -> ()  [unwired: 2 in, 2 out]
          }
          frame "Analog Out", "Motor", "PWM" {
            w261 = FALSE ("Visible")
            n137 = case shown="\"Analog Out\"" w260 {
              tunnel: [1.0 ("Value") -1.0 ("Value") 0.0 ("Value")] -> w259
              tunnel: [255.0 ("Value") 1.0 ("Value") 5.0 ("Value")] -> w258
              tunnel: [128.0 ("Value") 0.0 ("Value") 0.0 ("Value")] -> w257
              tunnel: [64.0 ("Value") 0.5 ("Value") 1.0 ("Value")] -> w256
              frame "PWM" {
              }
              frame "Motor", Default {
              }
              frame "Analog Out" {
              }
            }
            n138 = property on="Motor" class="Clust (strict)"("Visible"=TRUE) -> ()  [unwired: 2 in, 2 out]
            n139 = property on="Value" class="Slide (strict)"("Value"=w257, "Scale.Minimum"=w259, "Scale.Maximum"=w258, "Scale.Increment"=w256) -> ()  [unwired: 2 in, 2 out]
            n140 = property on="On/Off" class="Bool (strict)"("Visible"=w261) -> ()  [unwired: 2 in, 2 out]
            n141 = property on="Test Slider" class="Slide (strict)"("Visible"=w261) -> ()  [unwired: 2 in, 2 out]
            n142 = property on="Test Ring" class="Ring (strict)"("Visible"=w261) -> ()  [unwired: 2 in, 2 out]
            n143 = property on="Rev/Fwd" class="Clust (strict)"("Visible"=w261) -> ()  [unwired: 2 in, 2 out]
          }
          frame "Servo" {
            w277 = FALSE ("Visible")
            n144 = call <vilib>:"NT Read Number.vi"("Name"=w279) -> ("Numeric"=w278:dbl)  [unwired: 9 in, 1 out]
            n145 = property on="Test Slider" class="Slide (strict)"("Visible"=TRUE, "Scale.Maximum"=170.0 ("Scale.Range:Maximum")) -> ()  [unwired: 2 in, 2 out]
            n146 = local write "Test Slider"(w278) -> ()
            n147 = property on="Motor" class="Clust (strict)"("Visible"=w277) -> ()  [unwired: 2 in, 2 out]
            n148 = property on="Rev/Fwd" class="Clust (strict)"("Visible"=w277) -> ()  [unwired: 2 in, 2 out]
            n149 = property on="On/Off" class="Bool (strict)"("Visible"=w277) -> ()  [unwired: 2 in, 2 out]
            n150 = property on="Test Ring" class="Ring (strict)"("Visible"=w277) -> ()  [unwired: 2 in, 2 out]
          }
          frame "Relay", "Solenoid" {
            w280 = FALSE ("Visible")
            n151 = property on="Motor" class="Clust (strict)"("Visible"=w280) -> ()  [unwired: 2 in, 2 out]
            n152 = property on="Test Slider" class="Slide (strict)"("Visible"=w280) -> ()  [unwired: 2 in, 2 out]
            n153 = Search and Replace String(input string=w281, search string="/Value  **", replace string="/Direction") -> (result string=w287:string)  [unwired: 5 in, 3 out]
            n154 = property on="Test Ring" class="Ring (strict)"("Visible"=w280) -> ()  [unwired: 2 in, 2 out]
            n155 = call <vilib>:"NT Read String.vi"("Name"=w287) -> ("String"=w285:string)  [unwired: 9 in, 1 out]
            n156 = Equal?(x="Both directions", y=w285) -> (x = y?=w283:bool)
            n157 = Not(x=w283) -> (.not. x?=w284:bool)
            n158 = property on="Rev/Fwd" class="Clust (strict)"("Visible"=w283) -> ()  [unwired: 2 in, 2 out]
            n159 = property on="On/Off" class="Bool (strict)"("Visible"=w284, "Caption.Text"=w282) -> ()  [unwired: 2 in, 2 out]
          }
          frame "Compressor", "Digital Out" {
            w290 = FALSE ("Visible")
            # "Get direction and finish"
            n160 = property on="Motor" class="Clust (strict)"("Visible"=w290) -> ()  [unwired: 2 in, 2 out]
            n161 = property on="Test Slider" class="Slide (strict)"("Visible"=w290) -> ()  [unwired: 2 in, 2 out]
            n162 = property on="Test Ring" class="Ring (strict)"("Visible"=w290) -> ()  [unwired: 2 in, 2 out]
            n163 = property on="On/Off" class="Bool (strict)"("Visible"=TRUE, "Caption.Text"=w291) -> ()  [unwired: 2 in, 2 out]
            n164 = property on="Rev/Fwd" class="Clust (strict)"("Visible"=FALSE) -> ()  [unwired: 2 in, 2 out]
          }
          frame "Camera" {
            n165 = call <vilib>:"Get Last Path Segment.vi"("String in"=w298) -> ("String out"=w299:string)  [unwired: 10 in]
            n166 = property on="On/Off" class="Bool (strict)"("Visible"=FALSE) -> ()  [unwired: 2 in, 2 out]
            n167 = property on="Motor" class="Clust (strict)"("Visible"=FALSE) -> ()  [unwired: 2 in, 2 out]
            n168 = property on="Rev/Fwd" class="Clust (strict)"("Visible"=FALSE) -> ()  [unwired: 2 in, 2 out]
            n169 = case shown="\"White Balance  **\"" w299 {
              tunnel: w298 -> [w305 w314 w323 w332 w341 _ w347]
              tunnel: w297 -> [w303 w311 w320 w329 w338 _ _]
              frame "Size  **" {
                n170 = Index Array(array=w303) -> (element=w302:cluster{string[]})  [unwired: 1 in]
                n171 = call <vilib>:"NT Read String.vi"("Name"=w305) -> ("String"=w304:string)  [unwired: 9 in, 1 out]
                n172 = Unbundle(w302) -> (w300:string[])
                n173 = Match First String(2:w300, 3:w304) -> (0:w301:i32)  [unwired: 1 out]
                n174 = property on="Test Ring" class="Ring (strict)"("Value"=w301, "Strings []"=w300) -> ()  [unwired: 2 in, 2 out]
                n175 = property on="Test Ring" class="Ring (strict)"("Visible"=TRUE) -> ()  [unwired: 2 in, 2 out]
                n176 = property on="Test Slider" class="Slide (strict)"("Visible"=FALSE) -> ()  [unwired: 2 in, 2 out]
              }
              frame "White Balance  **" {
                n177 = Index Array(array=w311, index=1) -> (element=w312:cluster{string[]})
                n178 = call <vilib>:"NT Read String.vi"("Name"=w314) -> ("String"=w313:string)  [unwired: 9 in, 1 out]
                n179 = Unbundle(w312) -> (w309:string[])
                n180 = Match First String(2:w309, 3:w313) -> (0:w308:i32)  [unwired: 1 out]
                n181 = property on="Test Ring" class="Ring (strict)"("Value"=w308, "Strings []"=w309) -> ()  [unwired: 2 in, 2 out]
                n182 = property on="Test Ring" class="Ring (strict)"("Visible"=TRUE) -> ()  [unwired: 2 in, 2 out]
                n183 = property on="Test Slider" class="Slide (strict)"("Visible"=FALSE) -> ()  [unwired: 2 in, 2 out]
              }
              frame "Exposure  **" {
                n184 = Index Array(array=w320, index=2) -> (element=w321:cluster{string[]})
                n185 = call <vilib>:"NT Read String.vi"("Name"=w323) -> ("String"=w322:string)  [unwired: 9 in, 1 out]
                n186 = Unbundle(w321) -> (w317:string[])
                n187 = Match First String(2:w317, 3:w322) -> (0:w318:i32)  [unwired: 1 out]
                n188 = property on="Test Ring" class="Ring (strict)"("Value"=w318, "Strings []"=w317) -> ()  [unwired: 2 in, 2 out]
                n189 = property on="Test Ring" class="Ring (strict)"("Visible"=TRUE) -> ()  [unwired: 2 in, 2 out]
                n190 = property on="Test Slider" class="Slide (strict)"("Visible"=FALSE) -> ()  [unwired: 2 in, 2 out]
              }
              frame "Exposure Priority  **" {
                n191 = Index Array(array=w329, index=3) -> (element=w330:cluster{string[]})
                n192 = call <vilib>:"NT Read String.vi"("Name"=w332) -> ("String"=w331:string)  [unwired: 9 in, 1 out]
                n193 = Unbundle(w330) -> (w326:string[])
                n194 = Match First String(2:w326, 3:w331) -> (0:w327:i32)  [unwired: 1 out]
                n195 = property on="Test Ring" class="Ring (strict)"("Value"=w327, "Strings []"=w326) -> ()  [unwired: 2 in, 2 out]
                n196 = property on="Test Ring" class="Ring (strict)"("Visible"=TRUE) -> ()  [unwired: 2 in, 2 out]
                n197 = property on="Test Slider" class="Slide (strict)"("Visible"=FALSE) -> ()  [unwired: 2 in, 2 out]
              }
              frame "Color Enable  **" {
                n198 = Index Array(array=w338, index=4) -> (element=w339:cluster{string[]})
                n199 = call <vilib>:"NT Read String.vi"("Name"=w341) -> ("String"=w340:string)  [unwired: 9 in, 1 out]
                n200 = Unbundle(w339) -> (w335:string[])
                n201 = Match First String(2:w335, 3:w340) -> (0:w336:i32)  [unwired: 1 out]
                n202 = property on="Test Ring" class="Ring (strict)"("Value"=w336, "Strings []"=w335) -> ()  [unwired: 2 in, 2 out]
                n203 = property on="Test Ring" class="Ring (strict)"("Visible"=TRUE) -> ()  [unwired: 2 in, 2 out]
                n204 = property on="Test Slider" class="Slide (strict)"("Visible"=FALSE) -> ()  [unwired: 2 in, 2 out]
              }
              frame Default {
                n205 = property on="Test Ring" class="Ring (strict)"("Visible"=FALSE) -> ()  [unwired: 2 in, 2 out]
                n206 = property on="Test Slider" class="Slide (strict)"("Visible"=FALSE) -> ()  [unwired: 2 in, 2 out]
              }
              frame "Brightness  **", "Color Level  **", "Compression  **", "FPS  **", "Sharpness  **" {
                n207 = call <vilib>:"NT Read Number.vi"("Name"=w347) -> ("Numeric"=w346:dbl)  [unwired: 9 in, 1 out]
                n208 = local write "Test Slider"(w346) -> ()
                n209 = property on="Test Slider" class="Slide (strict)"("Visible"=TRUE, "Scale.Maximum"=100.0 ("Scale.Range:Maximum")) -> ()  [unwired: 2 in, 2 out]
                n210 = property on="Test Ring" class="Ring (strict)"("Visible"=FALSE) -> ()  [unwired: 2 in, 2 out]
              }
            }
          }
        }
        n211 = property on="Progress" class="Clust (strict)"("Visible"=FALSE) -> ()  [unwired: 2 in, 2 out]
      }
      event "Test Name": Mouse Enter {
        # "Populate the ring with the list of tests"
        n212 = event-data() -> ()  [unwired: 1 in, 1 out]
        n213 = call <vilib>:"NT Read String Array.vi"("Name"="TestMode/TestList") -> ("String Array"=w355:string[])  [unwired: 9 in, 1 out]
        n214 = Build Array (concatenate)("Select the test to run...", w355) -> (w354:string[])
        n215 = property on="Test Name" class="Ring (strict)"("Strings []"=w354) -> ()  [unwired: 2 in, 2 out]
      }
      event "Test Name": Value Change {
        w357 = FALSE ("Visible")
        # "Tell the robot the test name to run"
        n216 = event-data() -> ("NewVal"=w361:u16)  [unwired: 1 in]
        n217 = property on="Test Name" class="Ring (strict)"() -> ("Strings []"=w362:string[])  [unwired: 2 in, 2 out]
        n218 = local write "Progress"(T6 {"Test Progress"=0, "Test Progress Text"=""} ("Progress")) -> ()
        n219 = Index Array(array=w362, index=w361) -> (element=w360:string)
        n220 = call <vilib>:"NT Write String.vi"("String"=w360, "Name"="TestMode/TestName") -> ()  [unwired: 9 in, 1 out]
        n221 = property on="Progress" class="Clust (strict)"("Visible"=TRUE) -> ()  [unwired: 2 in, 2 out]
        n222 = property on="Motor" class="Clust (strict)"("Visible"=w357) -> ()  [unwired: 2 in, 2 out]
        n223 = property on="Test Slider" class="Slide (strict)"("Visible"=w357) -> ()  [unwired: 2 in, 2 out]
        n224 = property on="On/Off" class="Bool (strict)"("Visible"=w357) -> ()  [unwired: 2 in, 2 out]
        n225 = property on="Rev/Fwd" class="Clust (strict)"("Visible"=w357) -> ()  [unwired: 2 in, 2 out]
        n226 = property on="Test Ring" class="Ring (strict)"("Visible"=w357) -> ()  [unwired: 2 in, 2 out]
      }
      event "Select Auto": Mouse Enter {
        # "Populate the combo box with the list of autonomous options"
        n227 = event-data() -> ()  [unwired: 1 in, 1 out]
        n228 = call <vilib>:"NT Read String Array.vi"("Name"="Auto List") -> ("String Array"=w364:string[])  [unwired: 9 in, 1 out]
        n229 = property on="Select Auto" class="CmbBox"("Strings[]"=w364) -> ()  [unwired: 2 in, 2 out]
      }
      event "Select Auto": Value Change {
        # "User modified the Auto Selection. Write to NT variable so robot knows."
        n230 = event-data() -> ("NewVal"=w367:string)  [unwired: 1 in]
        n231 = call <vilib>:"NT Write String.vi"("String"=w367, "Name"="Auto Selector") -> ()  [unwired: 9 in, 1 out]
      }
      event "Command Selection": Value Change {
        # "Get the params and show in table"
        n232 = event-data() -> ("NewVal"=w373:i32)  [unwired: 1 in]
        n233 = property on="Command Selection" class="MCListbox (strict)"() -> ("ItemNames"=w371:string[][])  [unwired: 2 in, 2 out]
        n234 = call <vilib>:"WPI_DashboardUpdate Command Params.vi"("NewVal"=w373, "Commands"=w371, "Param Tbl"=w372) -> ()  [unwired: 8 in, 1 out]
      }
      event "Execute Command": Value Change {
        # "Started one, Unique ID holds\nresponse"
        n235 = event-data() -> ()  [unwired: 1 in, 1 out]
        n236 = property on="Command Selection" class="MCListbox (strict)"() -> ("ItemNames"=w384:string[][])  [unwired: 2 in, 2 out]
        n237 = Index Array(array=w384, index (row)="Command Selection", index (col)=0) -> (element=w382:string)
        n238 = call <vilib>:"Invoke Commands.vi"("Command Params"="Command Params", "Function Name"=w382) -> ("Params"=w378:u8, "Started"=w377:bool)  [unwired: 7 in, 1 out]
        n239 = Array Subset(array="Command Params", length (row)=w378) -> (w379:string[][])  [unwired: 3 in]
        n240 = Select(t="Executing" ("Cmd Status"), s=w377, f="" ("Cmd Status")) -> (s? t:f=→"Cmd Status":string)
      }
      event "Command Selection": Double Click {
        n241 = event-data() -> ("Row"=w392:i32)  [unwired: 1 in]
        n242 = property on="Command Selection" class="MCListbox (strict)"() -> ("ItemNames"=w395:string[][])  [unwired: 2 in, 2 out]
        n243 = local read "Command Params"() -> (w391:string[][])
        n244 = Index Array(array=w395, index (row)=w392, index (col)=0) -> (element=w393:string)
        n245 = call <vilib>:"Invoke Commands.vi"("Command Params"=w391, "Function Name"=w393) -> ("Params"=w390:u8, "Started"=w385:bool)  [unwired: 7 in, 1 out]
        n246 = Array Subset(array=w391, length (row)=w390) -> (w389:string[][])  [unwired: 3 in]
        n247 = Select(t="Executing" ("Cmd Status"), s=w385, f="" ("Cmd Status")) -> (s? t:f=w386:string)
        n248 = local write "Cmd Status"(w386) -> ()
      }
      event "CheckList": Double Click {
        # "Shift clears all"
        # "Update symbols on the listbox"
        n249 = event-data() -> ("PlatMods.Shift"=w397:bool, "Row"=w399:i32)  [unwired: 1 in]
        n250 = case shown="True" w397 {
          tunnel: w399 -> [w403 _]
          tunnel: 1 -> [w402 _]
          frame False {
            n251 = property on="CheckList" class="LstBox (strict)"() -> ("Item Symbols"=w401:i32[])  [unwired: 2 in, 2 out]
            n252 = Replace Array Subset(array=w401, new element=w402, index=w403) -> (w400:i32[])
            n253 = property on="CheckList" class="LstBox (strict)"("Item Symbols"=w400) -> ()  [unwired: 2 in, 2 out]
          }
          frame True {
            w404 = 0 ("Top Row")
            n254 = property on="CheckList" class="LstBox (strict)"() -> ("Number of Rows"=w406:u32)  [unwired: 2 in, 2 out]
            n255 = Initialize Array(0, w406) -> (w405:i32[])
            n256 = property on="CheckList" class="LstBox (strict)"("Top Row"=w404, "Value"=w404, "Item Symbols"=w405) -> ()  [unwired: 2 in, 2 out]
          }
        }
      }
      event "CheckList": Key Down {
        # "Update symbols on the listbox\nLeft and right keys check and uncheck"
        n257 = event-data() -> ("VKey"=w410:T21)  [unwired: 1 in]
        n258 = case shown="\"Left\", \"Right\"" w410 {
          selector: w410 -> [w415 _]
          tunnel: eventvkey."Left" ("VKey") -> [w413 _]
          frame "Left", "Right" {
            n259 = Equal?(x=w413, y=w415) -> (x = y?=w414:bool)
            n260 = Select(t=0, s=w414, f=1) -> (s? t:f=w416:i32)
            n261 = property on="CheckList" class="LstBox (strict)"() -> ("Item Symbols"=w419:i32[])  [unwired: 2 in, 2 out]
            n262 = Replace Array Subset(array=w419, new element=w416, index="CheckList") -> (w418:i32[])
            n263 = property on="CheckList" class="LstBox (strict)"("Item Symbols"=w418) -> ()  [unwired: 2 in, 2 out]
          }
          frame Default {
          }
        }
      }
      event "Motor.Enable": Value Change {
        # "When the test mode otor enable helper is set, update that\ntree row item's value"
        n264 = event-data() -> ("NewVal"=w425:bool)  [unwired: 1 in]
        n265 = Unbundle("Motor") -> ("Value"=w424:dbl)  [unwired: 1 out]
        n266 = Select(t=w424, s=w425, f=0.0) -> (s? t:f=w422:dbl)
        n267 = call <vilib>:"NT Write Number.vi"("Numeric"=w422, "Name"=w421) -> ()  [unwired: 9 in, 1 out]
      }
      event "Test Slider": Value Change {
        # "When the test mode slider helper is set, update that\ntree row item's value"
        n268 = event-data() -> ("NewVal"=w428:dbl)  [unwired: 1 in]
        n269 = call <vilib>:"NT Write Number.vi"("Numeric"=w428, "Name"=w429) -> ()  [unwired: 9 in, 1 out]
      }
      event "On/Off": Value Change {
        # "When the test mode on/off helper value is set, update that\ntree row item's value"
        n270 = event-data() -> ("NewVal"=w433:bool)  [unwired: 1 in]
        n271 = Boolean To (0,1)(Boolean=w433) -> (0, 1=w432:i16)
        n272 = call <vilib>:"NT Write Number.vi"("Numeric"=w432, "Name"=w431) -> ()  [unwired: 9 in, 1 out]
      }
      event "Rev/Fwd": Value Change {
        # "When the test mode helper value for relays is set, update that\ntree row item's value"
        n273 = event-data() -> ("NewVal.Forward"=w441:bool, "NewVal.Reverse"=w440:bool)  [unwired: 1 in]
        n274 = Boolean To (0,1)(Boolean=w441) -> (0, 1=w437:i16)
        n275 = Boolean To (0,1)(Boolean=w440) -> (0, 1=w439:i16)
        n276 = Negate(x=w439) -> (-x=w438:i16)
        n277 = Add(x=w437, y=w438) -> (x+y=w436:i16)
        n278 = call <vilib>:"NT Write Number.vi"("Numeric"=w436, "Name"=w435) -> ()  [unwired: 9 in, 1 out]
      }
      event "Test Ring": Value Change {
        # "When a test mode helper value is selected from the ring,\nset the tree item's variable to the string value"
        n279 = event-data() -> ("NewVal"=w445:u16)  [unwired: 1 in]
        n280 = property on="Test Ring" class="Ring (strict)"() -> ("Strings []"=w446:string[])  [unwired: 2 in, 2 out]
        n281 = Index Array(array=w446, index=w445) -> (element=w444:string)
        n282 = call <vilib>:"NT Write String.vi"("String"=w444, "Name"=w443) -> ()  [unwired: 9 in, 1 out]
      }
      event "Rec Mode": Value Change {
        # "Update globals for recording mode and path to read log from.\nClear when logging and let NetworkTables set path for vision to\nuse."
        n283 = event-data() -> ("NewVal"=w457:enum32{"Stop", "Record", "Playback"})  [unwired: 1 in]
        n284 = global write "WPI_DashboardLogging Global.vi" "Logging Filename"(path "") -> ()
        n285 = global write "WPI_DashboardLogging Global.vi" "Recording"(w457) -> ()
        n286 = case shown="\"Playback\"" w457 {
          tunnel: w456 -> [_ w459 w468]
          tunnel: [_ _ w467] -> w454
          tunnel: [_ _ w466] -> _
          tunnel: w452 -> [_ _ w464]
          tunnel: cluster{i32, i32} {-250, 170} -> [_ _ w463]
          tunnel: [_ _ T22 {"Image Size"=TRUE, "Image Type"=TRUE, "Pixel Value"=TRUE, "ROI Information"=TRUE, "Zoom Factor"=FALSE} ("Image Information Shown:All Elements")] -> w447
          tunnel: [_ _ TRUE ("Zoom Factor")] -> w448
          tunnel: w450 -> [_ _ w460]
          frame Default {
          }
          frame "Stop", "Record" {
            # "Place Window too"
            n287 = invoke class="VI" method="FP.Close"(reference=w459) -> (reference out=w458:refnum<vi>)  [unwired: 2 in, 2 out]
            n288 = invoke class="VI" method="Abort VI"(reference=w458) -> ()  [unwired: 2 in, 3 out]
          }
          frame "Playback" {
            n289 = call "Open Playback Panel.vi"("Offset"=w463, "DB VI Ref"=w464, "Playback in"=w468) -> ("Playback out"=w465:refnum<vi>)  [unwired: 8 in]
            n290 = register-events(w465, w460) -> (reference out=w467:refnum<event-registration>, error out=w466:errorcluster)  [unwired: 2 in]
          }
        }
        n291 = property on="Camera Image Right" class="ImageControl"("Image Information Shown"=w447, "Image Information Visible"=w448) -> ()  [unwired: 2 in, 2 out]
        n292 = property on="Camera Image" class="ImageControl"("Image Information Shown"=w447, "Image Information Visible"=w448) -> ()  [unwired: 2 in, 2 out]
        n293 = call <vilib>:"WPI_DashboardNT Log FieldName Cache.vi"("Operation"=enum16{"Lookup/Add", "Index", "Clear"}."Clear") -> ()  [unwired: 8 in, 3 out]
      }
      event Panel Close {
        w470 = enum32{"Stop", "Record", "Playback"}."Stop" ("Rec Mode")
        # "Playback window has been closed, abort"
        n294 = event-data() -> ()  [unwired: 1 in, 4 out]
        n295 = local write "Rec Mode"(w470) -> ()
        n296 = global write "WPI_DashboardLogging Global.vi" "Recording"(w470) -> ()
      }
      event Panel Close {
        # "Abort playback window and ourself"
        n297 = event-data() -> ()  [unwired: 1 in, 4 out]
        n298 = invoke class="VI" method="FP.Close"(reference=w474) -> (reference out=w473:refnum<vi>)  [unwired: 2 in, 2 out]
        n299 = invoke class="VI" method="Abort VI"(reference=w473) -> (error out=w472:errorcluster)  [unwired: 2 in, 2 out]
        n300 = invoke class="VI" method="Abort VI"(error in=w472) -> ()  [unwired: 2 in, 3 out]
      }
      event User Event {
        n301 = event-data() -> ("IDs"=w481:cluster{"RPC field ID":u16, "Unique ID":u16}, "String"=w480:string)  [unwired: 1 in]
        n302 = Bundle("IDs"=w481, "String"=w480) -> (w479:T9)  [unwired: 1 in]
        n303 = call <vilib>:"Retrieve RPC Response.vi"("RPC Response"=w479) -> ("Output"=w477:string[][])  [unwired: 10 in]
        n304 = Build Array (concatenate)(w475, w477) -> (w476:string[][])
        n305 = local write "Command Params"(w476) -> ()
        n306 = local write "Cmd Status"("" ("Cmd Status")) -> ()
      }
      event "Tree": Double Click {
        n307 = event-data() -> ("PlatMods"=w487:T25, "Tag"=w484:string)  [unwired: 1 in]
        n308 = Unbundle(w487) -> ("Shift"=w486:bool)  [unwired: 4 out]
        n309 = String Subset(string=w484, length (rest)=1 ("length (rest)")) -> (substring=w483:string)  [unwired: 1 in]
        n310 = Not(x=w486) -> (.not. x?=w485:bool)
        n311 = case shown="\"/\"" w483 {
          tunnel: w484 -> [_ w490]
          tunnel: w485 -> [_ w489]
          frame Default {
          }
          frame "/" {
            n312 = call <vilib>:"NT Update Persistence.vi"("Persistence"=w489, "Name"=w490) -> ()  [unwired: 9 in, 1 out]
          }
        }
      }
    }
  }
  n313 = Index Array(array=w72) -> (element=w70:refnum<vi>)  [unwired: 1 in]
  n314 = while {
    tunnel: w70 -> [w492]
    i -> [w495]
    stop <- FALSE stop-if-true
    n315 = Wait (ms)(milliseconds to wait=u32 100) -> ()  [unwired: 1 out]
    n316 = case shown="\"Playback\"" "Rec Mode" {
      tunnel: w495 -> [_ _ w510]
      tunnel: [u32 2829099 ("Base Color") u32 11141120 ("Target Color") w499] -> w491
      frame "Stop", Default {
        # "Reset the color, extra updates don't cost much"
      }
      frame "Record" {
      }
      frame "Playback" {
        # "Playback"
        n317 = Quotient & Remainder(x=w510, y=u32 50 ("milliseconds to wait")) -> (x-y*floor(x/y)=w506:u32)  [unwired: 1 out]
        n318 = Divide(x=w506, y=u32 50 ("milliseconds to wait")) -> (x/y=w503:dbl)
        n319 = Multiply(x=6.283185307179586, y=w503) -> (x*y=w508:dbl)
        n320 = Sine(x=w508) -> (sin(x)=w507:dbl)
        n321 = Absolute Value(x=w507) -> (abs(x)=w500:dbl)
        n322 = call "Interpolate RGB Color.vi"("Proportion"=w500, "Target Color"=u32 30976, "Base Color"=u32 2829099) -> ("Result Color"=w499:u32)  [unwired: 8 in]
      }
    }
    n323 = property class="Pane"(reference=w492, "PaneColor"=w491) -> ()  [unwired: 1 in, 2 out]
  }
  n324 = local write "Dashboard Tab"(T2."Drive" ("Dashboard Tab")) -> ()
  n325 = property on="On/Off" class="Bool (strict)"("Visible"=w41) -> ()  [unwired: 2 in, 2 out]
  n326 = property on="Motor" class="Clust (strict)"("Visible"=w41) -> ()  [unwired: 2 in, 2 out]
  n327 = property on="Progress" class="Clust (strict)"("Visible"=w41) -> ()  [unwired: 2 in, 2 out]
  n328 = property on="Test Ring" class="Ring (strict)"("Visible"=w41) -> ()  [unwired: 2 in, 2 out]
  n329 = property on="Rev/Fwd" class="Clust (strict)"("Visible"=w41) -> ()  [unwired: 2 in, 2 out]
  n330 = while {
    tunnel: u16 1741 ("timeout ms (25000)") -> [w512]
    stop <- FALSE stop-if-true
    n331 = TCP Create Listener(10:w512) -> (0:w511:errorcluster, 3:w513:refnum<k5>)  [unwired: 4 in, 1 out]
    n332 = case shown="No Error" w511 {
      selector: w511 -> [w515 _]
      tunnel: w513 -> [w516 _]
      frame No Error {
        n333 = while {
          tunnel: w516 -> [w519]
          tunnel: w515 -> [w518]
          stop <- FALSE stop-if-true
          n334 = TCP Wait On Listener(8:w518, 11:w519) -> (0:w520:errorcluster, 4:w521:refnum<k5>)  [unwired: 2 in, 3 out]
          n335 = local write "TCP"(w521) -> ()
          n336 = case shown="No Error" w520 {
            frame No Error {
            }
            frame Error {
              n337 = Wait (ms)(milliseconds to wait=u32 1000) -> ()  [unwired: 1 out]
            }
          }
        }
      }
      frame Error {
        n338 = Wait (ms)(milliseconds to wait=u32 1000) -> ()  [unwired: 1 out]
      }
    }
  }
  n339 = local write "Command Selection"(u16 0 ("milliseconds to wait")) -> ()
  n340 = local write "Command Params"(string[][] [] ("Command Params")) -> ()
  n341 = local write "Rec Mode"(w64) -> ()
  n342 = global write "WPI_DashboardLogging Global.vi" "Recording"(w64) -> ()
  n343 = call <vilib>:"NT Write String.vi"("String"="Select test", "Name"="Auto Selector") -> ()  [unwired: 9 in, 1 out]
  n344 = call-poly <vilib>:"NT Write Value.vi"("String"="Position", "Name"="Real_Pos") -> ()  [unwired: 9 in, 1 out]
  n345 = call-poly <vilib>:"NT Write Value.vi"("Boolean"="A second driver", "Name"="Second_Driver") -> ()  [unwired: 9 in, 1 out]
  n346 = call <vilib>:"WPI_DriverStationGame Specific Data.vi"() -> ("Game Specific Data"=w1:string)  [unwired: 11 in]
  n347 = local write "Game Data"(w1) -> ()
